vi "UI_guessLetter.vi"(8 "error in (no error)":errorcluster, 10 "buyingVowel?":bool) -> (0 "error out":errorcluster, 3 "Letter OUT":string)   [LabVIEW 2020]
panel:
  in  "Accept":bool
  in  "Letter":string caption="Consonant"
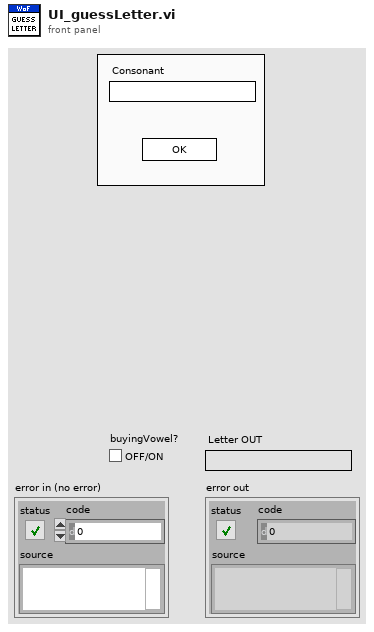
[diagram p1: front panel]
types:
  T1 = enum8{"Enabled", "Disabled", "Disabled and Grayed Out"}
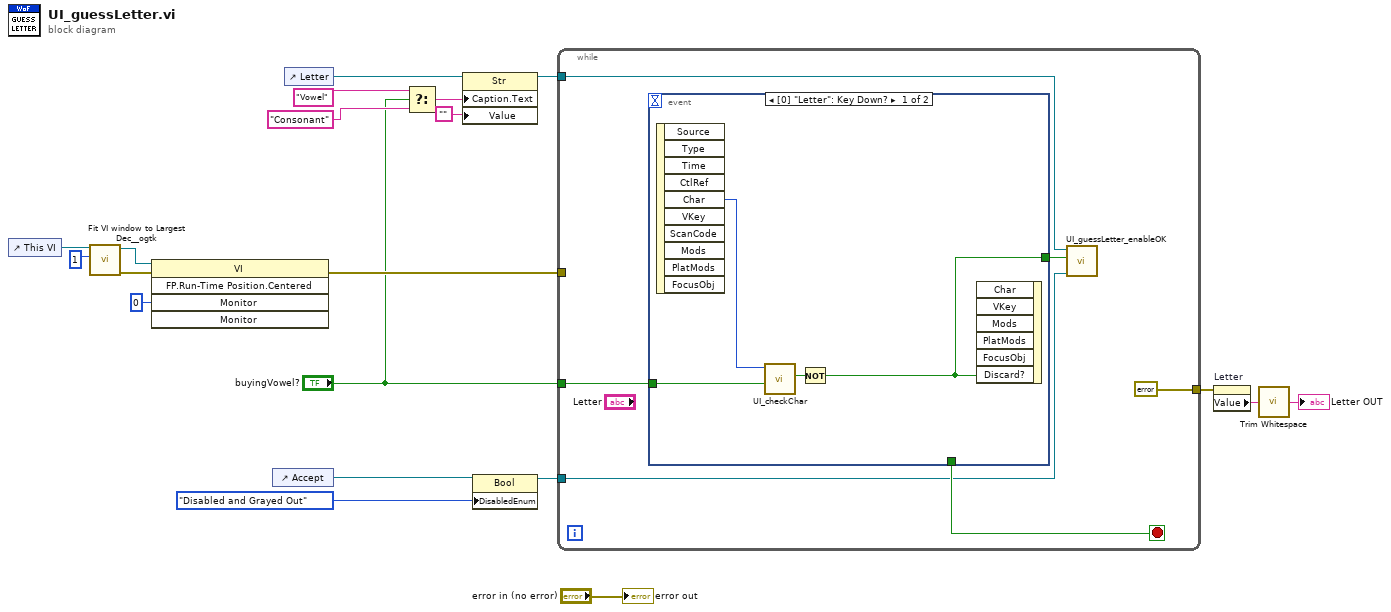
[diagram p0: block diagram]
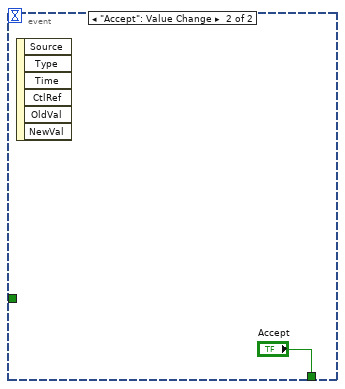
[diagram p2: hidden frame]
diagram:
  n1 = control-ref of="This VI"() -> (w9:refnum<vi>)
  n2 = call <userlib>:"Fit VI window to Largest Dec__ogtk.vi"("border spacing (2 px)"=1, "VI Ref (calling VI)"=w9) -> ("error out"=w5:errorcluster, "dup VI Ref"=w4:refnum<vi>)  [unwired: 4 in]
  n3 = invoke class="VI" method="FP.Run-Time Position.Centered"(reference=w4, error in=w5, "Monitor"=i16 0) -> (error out=w3:errorcluster)  [unwired: 2 in, 4 out]
  n4 = control-ref of="Accept"() -> (w18:refnum<vi>)
  n5 = control-ref of="Letter"() -> (w14:refnum<vi>)
  n6 = Select(t="Vowel", s="buyingVowel?", f="Consonant") -> (s? t:f=w10:string)
  n7 = property class="Str"(reference=w14, "Caption.Text"=w10, "Value"="") -> (reference out=w13:refnum<vi>)  [unwired: 1 in, 1 out]
  n8 = property class="Bool"(reference=w18, "DisabledEnum"=T1."Disabled and Grayed Out" ("Disabled")) -> (reference out=w16:refnum<vi>)  [unwired: 1 in, 1 out]
  n9 = while {
    tunnel: "buyingVowel?" -> [w26]
    tunnel: [errorcluster {"status"=FALSE, "code"=0, "source"=""} ("error in (no error)")] -> w20
    tunnel: w16 -> [w22]
    tunnel: w13 -> [w21]
    tunnel: w3 -> [_]
    stop <- w24 stop-if-true
    n10 = event shown="[0] \"Letter\": Key Down?" {
      selector: _ -> [_ _]
      dyn-events: _ -> [_ _]
      timeout: _ -> [_ _]
      tunnel: w26 -> [w29 _]
      tunnel: [_ "Accept"] -> w24
      tunnel: [w27 _] -> w23
      event "Letter": Key Down? {
        n11 = event-data() -> ("Char"=w30:i16)  [unwired: 1 in, 9 out]
        n12 = call "UI_checkChar.vi"("Buying Vowel?"=w29, "Char"=w30) -> ("Char OK?"=w28:bool)  [unwired: 9 in]
        n13 = Not(x=w28) -> (.not. x?=w27:bool)
        n14 = event-data("Discard?"=w27) -> ()  [unwired: 6 in, 1 out]
      }
      event "Accept": Value Change {
        n15 = event-data() -> ()  [unwired: 1 in, 6 out]
      }
    }
    n16 = call "UI_guessLetter_enableOK.vi"("Accept"=w22, "charDiscarded?"=w23, "Letter"=w21) -> ()  [unwired: 9 in]
  }
  n17 = property on="Letter" class="Str"(error in=w20) -> ("Value"=w19:string)  [unwired: 1 in, 2 out]
  n18 = call <vilib>:"Trim Whitespace.vi"("string"=w19) -> ("trimmed string"=→"Letter OUT":string)  [unwired: 1 in]
  "error out" <- "error in (no error)"
